vi "Extract Header Data Array.vi"(0 "Profile Data":u32[](array[numeric]), 5 "Profile Info":T1, 7 "Profile Index (0)":u32, 9 "Profile Cnt (0: rest)":u32, 11 "error in (no error)":errorcluster) -> (4 "Encoder Cnt Array":u32[](array[numeric]), 6 "Encoder Z-in Array":u32[](array[numeric]), 8 "Trigger Cnt Array":u32[](array[numeric]), 15 "error out":errorcluster)   [LabVIEW 8.6, in "Keyence LJ-V7000.lvlib"]
doc: "Only various data composing headers will be extracted to output in one dimensional array from profile data acquired with VI such as <B>Read Profiles (for High-Speed Mode)</B> VI.\n\n<B>Note</B>:\nRefer to <B>10.4</B> in a manual of measuring instrument drivers for profile headers.."
uses:
  Keyence LJ-V7000.lvlib
  Clusters/Profile Info.ctl
panel:
  out "Extract Cnt for Debug":u32
  # "(c) 2012 KEYENCE CORPORATION.  ALL RIGHTS RESERVED."
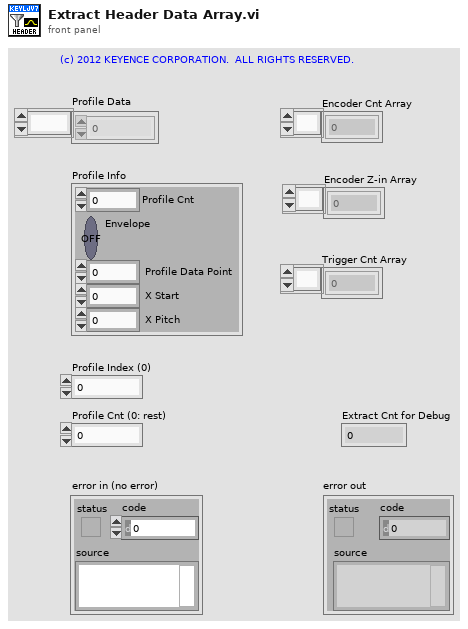
[diagram p1: front panel]
types:
  T1 = typedef "Keyence LJ-V7000.lvlib/Profile Info.ctl" = cluster{"Profile Cnt":u8, "Envelope":bool, " Profile Data Point":u16, " X Start":i32, " X Pitch":i32}
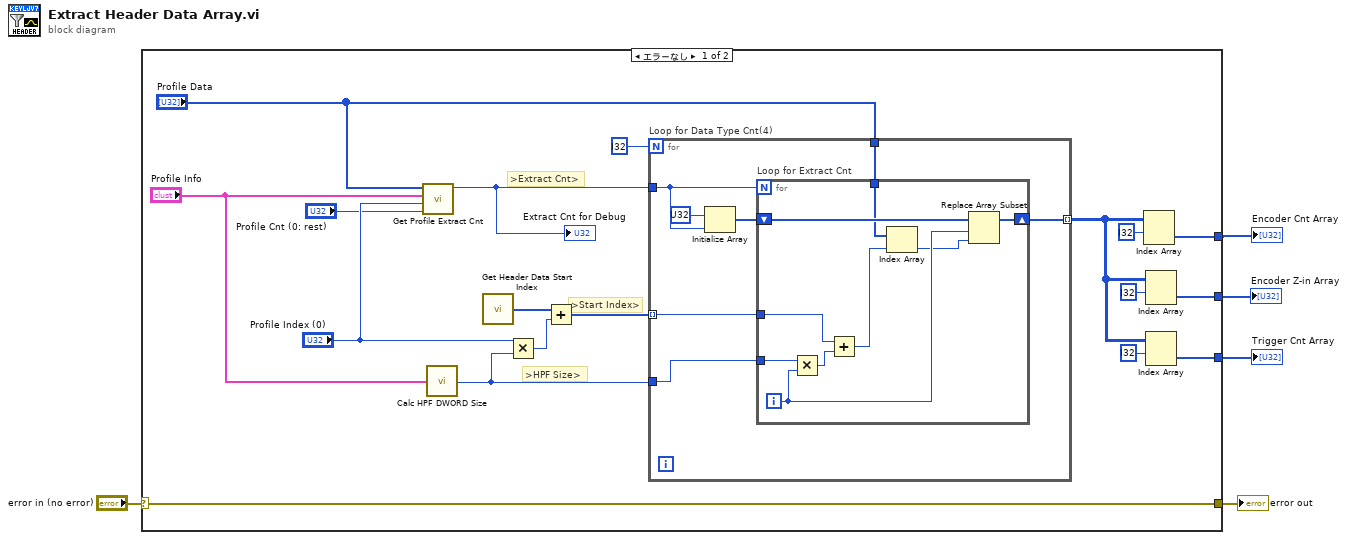
[diagram p0: block diagram]
diagram:
  n1 = case shown="エラーなし" "error in (no error)" {
    selector: "error in (no error)" -> [w11 w40]
    tunnel: [w17 _] -> w3
    tunnel: [w16 _] -> w2
    tunnel: [w13 _] -> w1
    tunnel: [w11 w40] -> w4
    frame #0 {
      # ">Start Index>"
      # ">Extract Cnt>"
      # ">HPF Size>"
      n2 = call "Get Profile Extract Cnt.vi"("Profile Cnt (0: rest)"="Profile Cnt (0: rest)", "Profile Index (0)"="Profile Index (0)", "Profile Info"="Profile Info", "Profile Data"="Profile Data") -> ("Extract Cnt"=w21:u32)  [unwired: 7 in]
      "Extract Cnt for Debug" <- w21
      n3 = call "Calc HPF DWORD Size.vi"("Profile Info"="Profile Info") -> ("DWORD Size"=w20:u32)  [unwired: 4 in]
      n4 = call "Get Header Data Start Index.vi"() -> ("Start Index[3]"=w10:u32[])  [unwired: 5 in]
      n5 = Multiply(x="Profile Index (0)", y=w20) -> (x*y=w19:u32)
      n6 = Add(x=w10, y=w19) -> (x+y=w22:u32[])
      n7 = for "Loop for Data Type Cnt(4)" {
        N: i32 ? -> [_]
        tunnel: w22 -> [w29] mode=indexing
        tunnel: w21 -> [w24]
        tunnel: w20 -> [w28]
        tunnel: [w27] -> w12 mode=indexing
        tunnel: "Profile Data" -> [w25]
        n8 = Initialize Array(u32 ?, w24) -> (w26:u32[])
        n9 = for "Loop for Extract Cnt" {
          N: w24 -> [_]
          tunnel: w29 -> [w37]
          tunnel: w28 -> [w39]
          shift-right: [w36] -> w27
          shift-left: w26 -> [w35]
          tunnel: w25 -> [w34]
          i -> [w32]
          n10 = Multiply(x=w39, y=w32) -> (x*y=w38:u32)
          n11 = Add(x=w37, y=w38) -> (x+y=w33:u32)
          n12 = Index Array(array=w34, index=w33) -> (element=w31:u32)
          n13 = Replace Array Subset(array=w35, new element=w31, index=w32) -> (w36:u32[])
        }
      }
      n14 = Index Array(array=w12, index (row)=i32 ? ("指標 （ページ）")) -> (element=w17:u32[])  [unwired: 1 in]
      n15 = Index Array(array=w12, index (row)=i32 ? ("指標 （ページ）")) -> (element=w16:u32[])  [unwired: 1 in]
      n16 = Index Array(array=w12, index (row)=i32 ? ("指標 （ページ）")) -> (element=w13:u32[])  [unwired: 1 in]
    }
    frame #1 {
    }
  }
  "error out" <- w4
  "Encoder Cnt Array" <- w3
  "Encoder Z-in Array" <- w2
  "Trigger Cnt Array" <- w1
